vi "Get Software Log Variables.vi"(8 "error in (no error)":errorcluster, 11 "LabVIEW Web Service Request":refnum<class "Web Request.lvclass">) -> (0 "error out":errorcluster, 3 "LabVIEW Web Service Request out":refnum<class "Web Request.lvclass">)   [LabVIEW 2018]
doc: "This VI sets all of the ESP variables for a single contact so it can be output from an ESP script."
uses:
  <vilib>/wsapi/Web Request.lvclass
  CAEN globals.vi
  <vilib>/wsapi/class/subVIs/Set Many String ESP Variables.vi
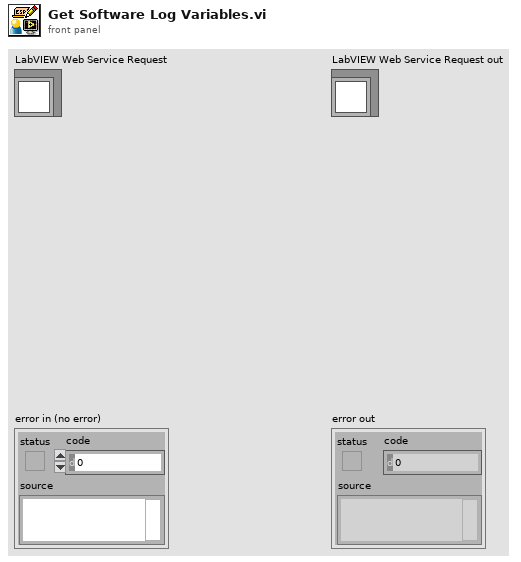
[diagram p1: front panel]
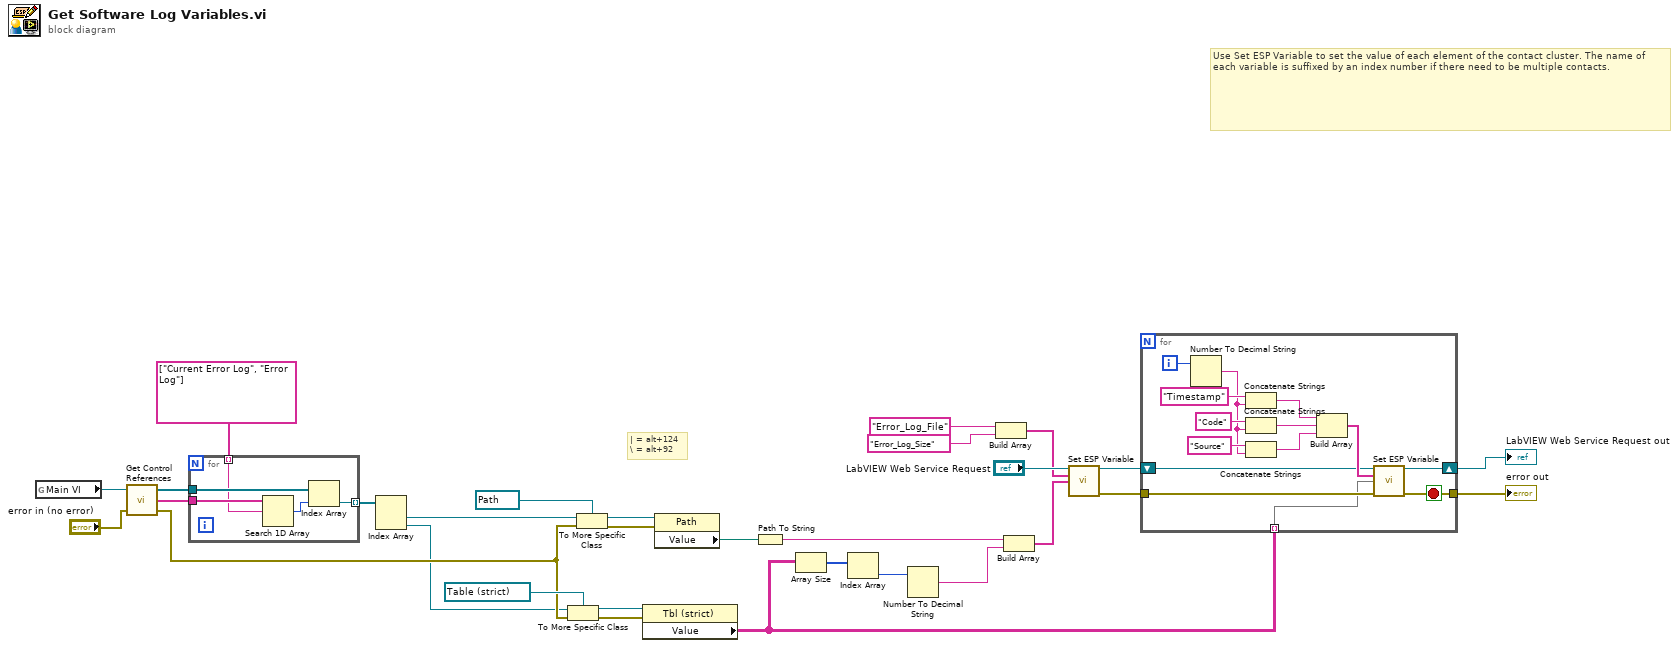
[diagram p0: block diagram]
diagram:
  # "| = alt+124\n\\ = alt+92"
  # "Use Set ESP Variable to set the value of each element of the contact cluster. The name of each variable is suffixed by an index number if there need to be multiple contacts."
  n1 = global read "CAEN globals.vi" "Main VI"() -> (w25:refnum<vi>)
  n2 = call "Get Control References.vi"("error in"="error in (no error)", "This vi"=w25) -> ("error out"=w15:errorcluster, "Control Names"=w24:string[], "Controls[]"=w23:refnum<vi>[])  [unwired: 1 in]
  n3 = for {
    tunnel: w24 -> [w35]
    tunnel: w23 -> [w33]
    tunnel: [w32] -> w20 mode=indexing
    tunnel: string[] ["Current Error Log", "Error Log"] ("Control Names") -> [w31] mode=indexing
    n4 = Search 1D Array(1D array=w35, element=w31) -> (index of element=w34:i32)  [unwired: 1 in]
    n5 = Index Array(array=w33, index=w34) -> (element=w32:refnum<vi>)
  }
  n6 = Index Array(array=w20) -> (element #1=w14:refnum<vi>, element #2=w13:refnum<vi>)  [unwired: 2 in]
  n7 = To More Specific Class(target class=refnum<vi> refnum ("Alarm Log"), reference=w13, error in=w15) -> (specific class reference=w19:refnum<vi>, error out=w18:errorcluster)
  n8 = To More Specific Class(target class=refnum<vi> refnum ("Current Error Log"), reference=w14, error in=w15) -> (specific class reference=w12:refnum<vi>, error out=w11:errorcluster)
  n9 = property class="Tbl (strict)"(reference=w19, error in=w18) -> ("Value"=w1:string[][])  [unwired: 2 out]
  n10 = property class="Path"(reference=w12, error in=w11) -> ("Value"=w10:path)  [unwired: 2 out]
  n11 = Path To String(path=w10) -> (string=w9:string)
  n12 = Array Size(array=w1) -> (size(s)=w4:i32[])
  n13 = Index Array(array=w4) -> (element=w3:i32)  [unwired: 1 in]
  n14 = Number To Decimal String(number=w3) -> (decimal integer string=w2:string)  [unwired: 1 in]
  n15 = Build Array("Error_Log_File" ("string"), "Error_Log_Size" ("string")) -> (w29:string[])
  n16 = Build Array(w9, w2) -> (w28:string[])
  n17 = call-poly <vilib>:"Set ESP Variable.vi"("LabVIEW Web Service Request"="LabVIEW Web Service Request", "keys"=w29, "values"=w28) -> ("LabVIEW Web Service Request out"=w8:refnum<class "Web Request.lvclass">, "error out"=w7:errorcluster)  [unwired: 11 in]
  n18 = for {
    tunnel: w7 -> [w49]
    tunnel: [w39] -> w6
    shift-right: [w40] -> w5
    shift-left: w8 -> [w42]
    tunnel: w1 -> [w36] mode=indexing
    i -> [w38]
    stop <- w39 stop-if-true
    n19 = Number To Decimal String(number=w38) -> (decimal integer string=w37:string)  [unwired: 1 in]
    n20 = Concatenate Strings("Timestamp" ("string"), w37) -> (w41:string)
    n21 = Concatenate Strings("Code" ("string"), w37) -> (w45:string)
    n22 = Concatenate Strings("Source" ("string"), w37) -> (w44:string)
    n23 = Build Array(w41, w45, w44) -> (w43:string[])
    n24 = call-poly <vilib>:"Set ESP Variable.vi"("LabVIEW Web Service Request"=w42, "keys"=w43, "values"=w36, "error in (no error)"=w49) -> ("LabVIEW Web Service Request out"=w40:refnum<class "Web Request.lvclass">, "error out"=w39:errorcluster)  [unwired: 10 in]
  }
  "error out" <- w6
  "LabVIEW Web Service Request out" <- w5
